vi "sub_single-cycle-config.vi"(9 "Single sequence":T1) -> ()   [LabVIEW 2019]
uses:
  sequence_single.ctl
  _ctrl/rw.ctl
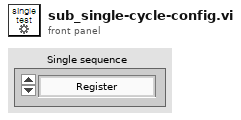
[diagram p1: front panel]
types:
  T1 = typedef "sequence_single.ctl" = enum16{"Register", "RC", "B1", "B2", "B3", "Oper_LV", "Oper_HV", "ContR_LV"}
  T2 = typedef "rw.ctl" = enum16{"read", "write"}
  T3 = typedef "ui_dev-operator.ctl" = cluster{"Operation stutus":refnum<vi>, "Test Status":refnum<vi>, "Setting":refnum<vi>, "Manual":refnum<vi>, "Main":refnum<vi>, "RCstart":refnum<vi>, "채널선택":refnum<vi>, "시험명":refnum<vi>, "Tab Control_manual":refnum<vi>, "시험 모드":refnum<vi>, "HW check":refnum<vi>, "login":refnum<vi>, "logout":refnum<vi>}
  T4 = typedef "Testing-info.ctl" = cluster{"전체채널수":u8, "현재채널번호":u8, "Irms":dbl, "입력전압":dbl, "입력전류":dbl, "출력전압":dbl, "출력전류":dbl, "온도":dbl, "제어단 단선":bool, "제어단 단락":bool, "제어단 특성변화":bool, "출력단 단선":bool, "출력단 단락":bool, "출력단 특성변화":bool, "출력단 전압":bool, "카운트 일치":bool, "Irms 판정":bool, "온도":bool, "테스트 회수":u32, "TestType":T1, "현재회수":u32, "Ch selection":cluster{"1ch":bool, "2ch":bool, "3ch":bool, "4ch":bool, "5ch":bool, "6ch":bool}, "반복":u32, "Path":path, "파일생성주기":u32, "start time":dbl, "stop time":dbl, "현재반복회수":u32, "NG":cluster{"입출력 카운트":bool, "출력전류RMS":bool}}
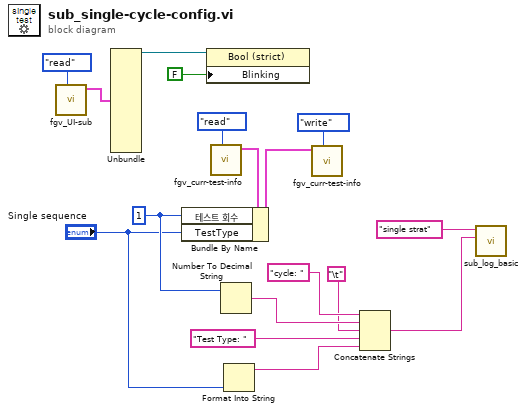
[diagram p0: block diagram]
diagram:
  w8 = u32 1 ("테스트 회수")
  n1 = call "fgv_UI-sub.vi"("cmd"=rw."read") -> ("output cluster 2"=w15:T3)  [unwired: 9 in, 1 out]
  n2 = Unbundle(w15) -> ("Operation stutus"=w14:refnum<vi>)  [unwired: 12 out]
  n3 = property class="Bool (strict)"(reference=w14, "Blinking"=FALSE) -> ()  [unwired: 1 in, 2 out]
  n4 = call "fgv_curr-test-info.vi"("cmd"=rw."read") -> ("현재테스트 정보 2"=w10:T4)  [unwired: 10 in]
  n5 = Bundle By Name(cluster=w10, "테스트 회수"=w8, "TestType"="Single sequence") -> (w9:T4)
  n6 = Number To Decimal String(number=w8) -> (decimal integer string=w6:string)  [unwired: 1 in]
  n7 = Format Into String("Single sequence") -> (resulting string=w3:string)  [unwired: 3 in, 1 out]
  n8 = call "fgv_curr-test-info.vi"("cmd"=rw."write", "현재테스트 정보"=w9) -> ()  [unwired: 9 in, 1 out]
  n9 = Concatenate Strings("cycle: " ("string"), w6, "\t", "Test Type: " ("string"), w3) -> (w2:string)
  n10 = call "sub_log_basic.vi"("desc"=w2, "Title"="single strat") -> ()  [unwired: 9 in, 1 out]
